vi "GetHisto.vi"   [LabVIEW 2014]
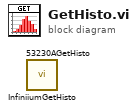
[diagram p0: block diagram]
diagram:
  n1 = call "InfiniiumGetHisto.vi"() -> ()  [unwired: 3 in, 1 out]
  n2 = call "53230AGetHisto.vi"() -> ()  [unwired: 3 in, 1 out]
